vi "testParseArguments.vi"(8 "error in (no error)":errorcluster, 11 "testStateMachineUtilities in":refnum<class "testStateMachineUtilities.lvclass">) -> (0 "error out":errorcluster, 3 "testStateMachineUtilities out":refnum<class "testStateMachineUtilities.lvclass">)   [LabVIEW 2013, in "testStateMachineUtilities.lvclass"]
uses:
  testStateMachineUtilities.lvclass
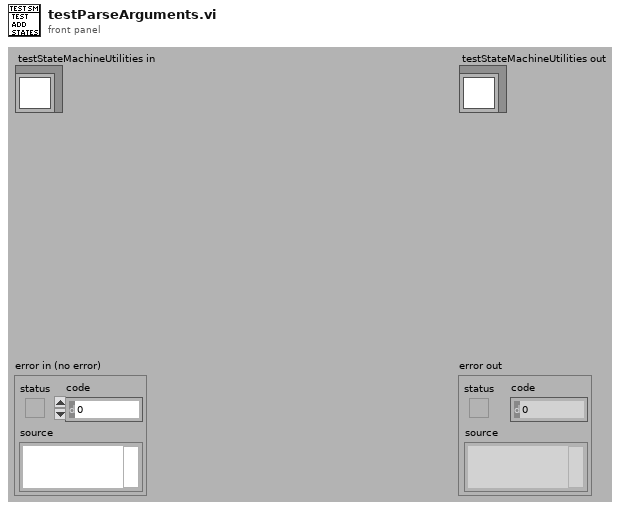
[diagram p1: front panel]
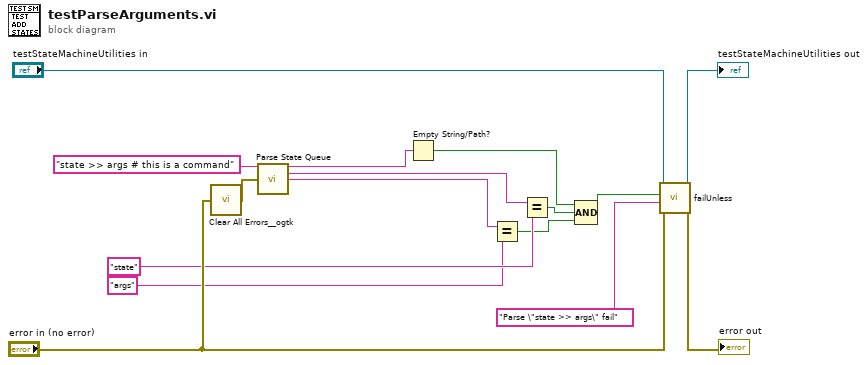
[diagram p0: block diagram]
diagram:
  n1 = call <userlib>:"Clear All Errors__ogtk.vi"("Error In"="error in (no error)") -> ("Error Out"=w11:errorcluster)  [unwired: 3 in]
  n2 = call "Parse State Queue.vi"("State Queue"="state >> args # this is a command", "Error In (no error)"=w11) -> ("Remaining States"=w2:string, "Current State"=w4:string, "Arguments"=w3:string)  [unwired: 10 in, 1 out]
  n3 = Empty String/Path?(string/path=w2) -> (empty?=w1:bool)
  n4 = Equal?(x=w3, y="args" ("State Queue")) -> (x = y?=w7:bool)
  n5 = Equal?(x=w4, y="state" ("State Queue")) -> (x = y?=w8:bool)
  n6 = Compound Arithmetic op=AND(w1, w8, w7) -> (w6:bool)
  n7 = call-dynamic "failUnless.vi"("error in (no error)"="error in (no error)", "message (\"\")"="Parse \"state >> args\" fail" ("message (\"\")"), "pass"=w6, "TestCase in"="testStateMachineUtilities in") -> ("error out"=→"error out":errorcluster, "TestCase out"=→"testStateMachineUtilities out":refnum<class "testStateMachineUtilities.lvclass">)  [unwired: 6 in]
